vi "SeriellRead.vi"(6 "SkalierungsfaktorHorst":dbl[](array[numeric]), 7 "VorwortHorst":string[](array[string]), 9 "Zwischenspeicher":string[](array[string]), 10 "Senden?":bool[](array[boolean]), 11 "FPGA VI Reference In":refnum<k20>) -> (1 "Senden?":bool[](array[boolean]), 2 "Zwischenspeicher":string[](array[string]))   [LabVIEW 2010]
uses:
  <vilib>/rvi/interface/nirviMethod/nirviMethod.xnode
  C:/Users/HAGAR-IV/Desktop/Zeugs/markus/version feb 2012/FPGA Bitfiles/pertrasgcfpga2_FPGATarget_FPGA-Programm-10_16368CB6.lvbitx
  C:/Users/HAGAR-IV/Desktop/Zeugs/Johnny/pertrasgc fpga/FPGA-Programm-10-14.vi
  <vilib>/rvi/interface/common/niFpgaNodeNameForErrorReporting.ctl
  <vilib>/rvi/errors/niLvFpgaWhatHappensToTopLevelVI.ctl
  <vilib>/Utility/error.llb/Error Cluster From Error Code.vi
  <vilib>/rvi/errors/niLvFpgaAdjustHostInterfaceError.vi
  GVStringArray.vi
  GVECDs.vi
  NiFpgaLv.dll
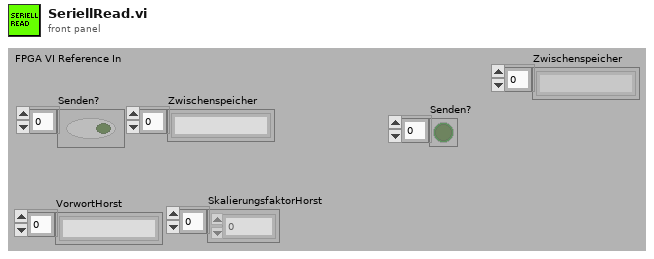
[diagram p1: front panel]
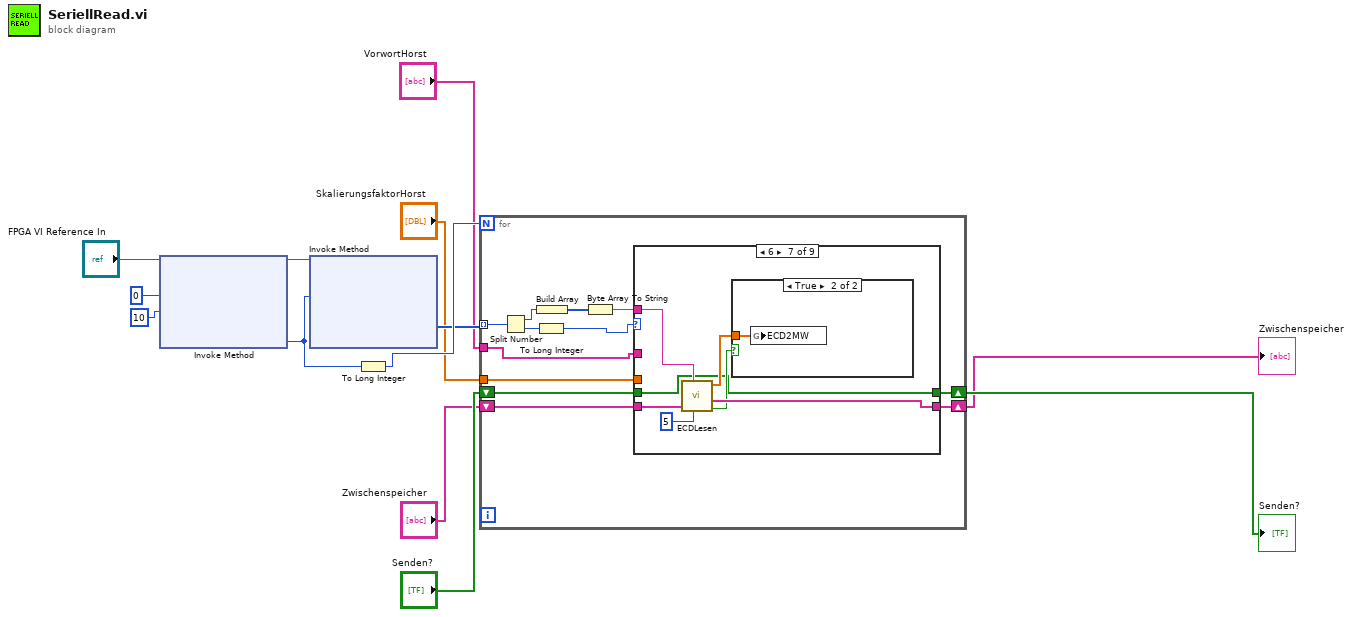
[diagram p0: block diagram]
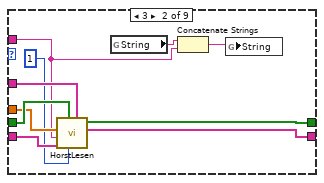
[diagram p3: hidden frame]
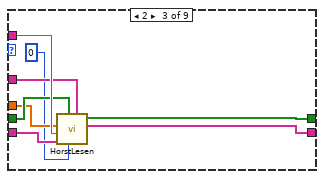
[diagram p4: hidden frame]
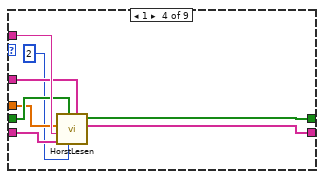
[diagram p5: hidden frame]
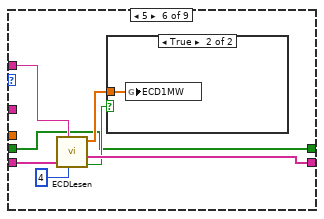
[diagram p7: hidden frame]
diagram:
  n1 = xnode "Invoke Method"("FPGA VI Reference In"="FPGA VI Reference In", "Number of Elements"=u32 0, "Timeout (ms)"=10) -> ("FPGA VI Reference Out"=w9:refnum<k20>, "Elements Remaining"=w12:u32)  [unwired: 1 in, 2 out]
  n2 = xnode "Invoke Method"("FPGA VI Reference In"=w9, "Number of Elements"=w12) -> ("Data"=w8:u16[])  [unwired: 2 in, 3 out]
  n3 = To Long Integer(number=w12) -> (32bit integer=w13:i32)
  n4 = for {
    N: w13 -> [_]
    tunnel: w8 -> [w25] mode=indexing
    shift-right: [w21] -> w4
    shift-left: "Senden?" -> [w20]
    shift-right: [w22] -> w3
    shift-left: "Zwischenspeicher" -> [w23]
    tunnel: "VorwortHorst" -> [w16]
    tunnel: "SkalierungsfaktorHorst" -> [w15]
    n5 = Split Number(x=w25) -> (hi(x)=w19:u8, lo(x)=w17:u8)
    n6 = To Long Integer(number=w17) -> (32bit integer=w14:i32)
    n7 = Build Array(w19) -> (w18:u8[])
    n8 = Byte Array To String(unsigned byte array=w18) -> (string=w24:string)
    n9 = case shown="6" w14 {
      tunnel: w24 -> [_ w29 w45 w53 _ w62 w70 _ _]
      tunnel: w23 -> [w27 w37 w44 w52 w55 w61 w69 w72 w74]
      tunnel: [w27 w36 w43 w51 w55 w60 w68 w72 w74] -> w22
      tunnel: [w26 w35 w42 w50 w54 w56 w64 w73 w75] -> w21
      tunnel: w20 -> [w26 w34 w41 w49 w54 w56 w64 w73 w75]
      tunnel: w16 -> [_ w33 w40 w48 _ _ _ _ _]
      tunnel: w15 -> [_ w32 w39 w47 _ _ _ _ _]
      frame 0, Default {
      }
      frame 3 {
        n10 = call "HorstLesen.vi"("VorwortHorst"=w33, "Port"=1, "Senden?"=w34, "Zwischenspeicher"=w37, "string"=w29, "SkalierungsfaktorHorst"=w32) -> ("Zwischenspeicher"=w36:string[], "Senden?"=w35:bool[])  [unwired: 4 in]
        n11 = global read "GVStringArray.vi" "String"() -> (w30:string)
        n12 = Concatenate Strings(w30, w29) -> (w28:string)
        n13 = global write "GVStringArray.vi" "String"(w28) -> ()
      }
      frame 2 {
        n14 = call "HorstLesen.vi"("VorwortHorst"=w40, "Port"=0, "Senden?"=w41, "Zwischenspeicher"=w44, "string"=w45, "SkalierungsfaktorHorst"=w39) -> ("Zwischenspeicher"=w43:string[], "Senden?"=w42:bool[])  [unwired: 4 in]
      }
      frame 1 {
        n15 = call "HorstLesen.vi"("VorwortHorst"=w48, "Port"=2, "Senden?"=w49, "Zwischenspeicher"=w52, "string"=w53, "SkalierungsfaktorHorst"=w47) -> ("Zwischenspeicher"=w51:string[], "Senden?"=w50:bool[])  [unwired: 4 in]
      }
      frame 4 {
      }
      frame 5 {
        n16 = call "ECDLesen.vi"("string"=w62, "Zwischenspeicher"=w61, "Port"=4) -> ("ECDMW"=w58:dbl[], "Zwischenspeicher"=w60:string[], "ECDEmpfangen?"=w59:bool)  [unwired: 3 in]
        n17 = case shown="True" w59 {
          tunnel: w58 -> [_ w63]
          frame False {
          }
          frame True {
            n18 = global write "GVECDs.vi" "ECD1MW"(w63) -> ()
          }
        }
      }
      frame 6 {
        n19 = call "ECDLesen.vi"("string"=w70, "Zwischenspeicher"=w69, "Port"=5) -> ("ECDMW"=w66:dbl[], "Zwischenspeicher"=w68:string[], "ECDEmpfangen?"=w67:bool)  [unwired: 3 in]
        n20 = case shown="True" w67 {
          tunnel: w66 -> [_ w71]
          frame False {
          }
          frame True {
            n21 = global write "GVECDs.vi" "ECD2MW"(w71) -> ()
          }
        }
      }
      frame 7 {
      }
      frame 8 {
      }
    }
  }
  "Senden?" <- w4
  "Zwischenspeicher" <- w3
